vi "ScopeIntegrateSignal.vi"() -> ()   [LabVIEW 2018]
doc: "This example illustrates how to use autosetup and continuously acquires waveforms from a single channel using the following steps:\n\n1. Specify a valid VISA session. \n2. Specify a channel. \n3. Specify a time-out value for reading waveform.\n4. Run the VI. The graph displays the waveform you acquire."
uses:
  <vilib>/Analysis/baseanly.llb/Mean (DBL).vi
  <vilib>/Analysis/8numeric.llb/1D Numeric Integration.vi
  <instrlib>/Tektronix DPO MSO 2000 4000 Series/Public/Data/Read (Single Waveform).vi
  <instrlib>/Tektronix DPO MSO 2000 4000 Series/Tektronix DPO MSO 2000 4000 Series.lvlib
  <vilib>/Analysis/NI_AALPro.lvlib
  <vilib>/Analysis/NI_AALBase.lvlib
panel:
  out "Numeric":i32=1328
  out "standard deviation":dbl=1.3029024695657787 format="%0.2f"
  out "mean":dbl=2.2899697361108426 format="%0.2f"
  in  "Looping?":bool=TRUE
  in  "stop":bool
  out "integrated signal array":dbl[](array[numeric])=[0.18384399999980483, 1.0317809999998684, 1.3195783888887622, 2.3158365555554963, 0.04278729777806473, 1.1630631999997754, 3.3124563999997245, 3.497783541110766, 3.1549023744437497, 3.755903906666071, 3.3056046966661468, 3.106938013333607, 2.0850505944443567, 0.7116690033303827, 0.3406699844465184, 0.2005544977782775, 0.8526708144434995, 17.02474333444437, 1.3222985777702674, 1.0146186222293065, 0.6997047444517787, 1.2871290444375227, 20.821349922229718, 0.5246940888823304, 2.799625122228476, 1.648999088882956, 0.1761865444374138, 1.4400063555625282, 0.4872134555622556, 0.182366488894913, 0.13585464445012588, 1.4629045222283865, 1.8308287333288202, 1.3392077333367414, 2.7180222222237846, 1.4216097111038173, 0.2816763222150883, 0.3812891444506439, 2.365242422216168, 2.3021390333392304, 0.6825071333286256, 0.0959767555478045, 1.0579274000075247, 0.4138698333410148, 1.304622111118793, 0.49093292221467383, 0.9457530444370531, 101.81548561111937, 1.529317866658801, 0.33561907777122146, 1.0599211333392058, 0.8035876777852327, 0.5726897111173316, 0.06260372221603036, 2.2174570111179697, 0.5724496666644885, 0.5157550999971418, 2.8346701888819488, 2.778916566673187, 0.765314000007485, 0.9394557555628589, 0.6897417333308761, 3.7532666666722387, 2.173821266666129, 0.4845779333312618, 1.060541600000534, 2.2861999333331147, 0.11699586666738315, 0.9563122888909481, 1.8866587555542365, 2.7708600444424665, 3.598289155551745, 1.7618008444416102, 1.1966221111136597, 2.265614066664132, 0.20330315555749479, 0.12547351111451932, 0.3422101111106736, 0.5313641333342627, 1.0522981555572077, 0.3378435777794101, 2.006787177780507, 2.1922246888884085, 3.361183577780303, 0.6140928222222171, 1.4745631555535357, 0.3275447555555265, 0.6753259555530603, 2.815404511113747, 0.44156842222977544, 1.689486888890445, 1.640821333334569, 2.9290531555559047, 0.6118766222224593, 151.72732157777253, 0.826040555558351, 2.2798071111146094, 0.36612853333442347, 1.370790888899429, 2.277512288885853, 2.583507888883297, 0.5587739999998309, 1.7333380222304962, 0.9870752666637039, 0.14599966667146197, 1.835137177779994, 0.23406471110102162, 0.49785124444643347, 0.5946523500004227, 0.07523338888929976, 0.5758768055563855, 0.0733093944444089, 0.359282266667846, 0.010280066666889544, 0.681827916665766, 0.3919141444447414, 0.12973324444464956, 0.6164764222229102, 0.3204300611109303, 0.0720933000008443, 0.12928820555576342, 0.6098657666660594, 0.11357656111182071, 0.26238870555593635, 0.37584263333213874, 0.2554021388892921, 0.20303043333085263, 0.3101077888884636, 0.35926910555497565, 0.00022648888919396017, 0.26812556111169467, 0.10511678333299901, 0.5440186111114619, 0.01743401111172833, 0.3281956277780249, 0.8202786388912735, 0.3696199722241836, 0.04841992222217021, 0.3239199111107238, 0.3001403277771748, 0.08190676111082815, 0.40686790555485663, 86.0430172333338, 0.0016486000007947049, 0.14501810000032683, 0.3358190111111883, 0.030844705554956643, 0.5548646833340989, 0.3074427111109858, 0.1855340222226348, 0.0023650388895090843, 0.5550829666656036, 0.3319229277786019, 0.2979634833328052, 0.6956377888881221, 0.4173154666666514, 0.6801122888883514, 0.139358950000252, 0.2027275388881625, 0.4752827277773105, 0.06920137222224754, 0.1462285888899195, 0.3104269499993294, 0.6071250944441561, 0.15783686666638486, 0.3827724055561009, 0.024903588888977986, 0.9917656444440512, 0.250505066669551, 0.10083276666760904, 0.37267306666646277, 0.34872057222288716, 0.5987366722238008, 0.6558884666666526, 0.0029425500005292034, 1.4289747000062263, 1.077603833340331, 0.2976313222159524, 0.16553077777104885, 0.04071188888223318, 0.6158996666579656, 0.6296267222305018, 0.0043566777700086495, 2.304217255548706, 1.149385477774478, 0.37190994443622916, 1.321093977771371, 0.8237574666736233, 0.4398182000074706, 0.34472841110549224, 101.6373810333415, 0.842691444459666, 4.352914222217547, 3.4642069999796674, 0.6703112222367144, 1.9725337222045751, 3.6376435555696567, 3.5489517222082103, 6.32480072220843, 6.1287116110974, 1.546892722234429, 5.2348347777493744, 1.0970715000174573, 6.749840833347956, 9.231031055566662, 3.8409967777967826, 1.4225064444326108, 2.374212277792598, 4.324341611124469, 2.3102265555462838, 5.294125333340804, 6.662379777792693, 1.101190333327366, 5.148103777766739, 11.361353666678252, 5.932165388874546, 8.079377111096475, 5.080487277791736, 7.687094111125154, 0.3043856111193732, 10.670411777788116, 10.065965944451424, 0.5244318333399753, 13.074301777792584, 5.415608833316831, 1.9877505555598742, 1.3460380222320463, 0.5223974444430709, 2.1154885555578624, 2.5680954444446416, 1.317197888891957, 1.7756387999954955, 0.6476903333353883, 2.000213466674835, 0.0013438888889201112, 0.6318706222236417, 0.3013760666611618, 25.54041106667208, 0.3399827111113684, 0.16931690555602244, 0.3304252166661164, 0.16594397222185006, 0.12300538333289182, 0.2824761944441453, 0.17886768888885446, 0.6391234222220713, 0.3861981777783553, 0.09919301111110637, 0.2602778944443442, 0.13828761666639436, 0.1439515499997701, 0.3348733555558696, 0.06759907222323568, 0.5780929555568003, 0.24132427777802898, 0.04788488333396096, 0.3549457666659056, 0.3813597611109805, 0.11640393888960737, 0.5092426666667609, 0.13405288888820138, 14.625359033335016, 0.05221748888888154, 0.31403203888894826, 0.6693128444436998, 0.005222283332966806, 0.3896295277778545, 0.7952144388883583, 0.24450921666717135, 0.5297790777771815, 0.20670765000030916, 0.5681828666660081, 0.1069472055550931, 0.13426145555557506, 0.3312466500002883, 0.43531609444513375, 0.11154298888868011, 0.2259397222227168, 0.1524273555549207, 0.24677374444440603, 0.09216521111142176, 0.3101080833340964, 0.22031912777769935, 0.2475422000001521, 1.3618345499998947, 17.445979400003228, 16.615822750000493, 0.4773475000002133, 0.3393787500008643, 0.04931600000073315, 0.12953424999985447, 0.28308700000064296, 0.19237174999942008, 0.5199734999998644, 0.142788500000246, 0.33203175000057883, 0.4310394999999665, 0.3645760000005205, 0.06618225000005556, 0.44678924999943687, 0.024376499999411837, 0.20625500000275016, 0.08267749999828847, 0.22802799999867632, 0.07276249999920412, 0.44335200000030284, 0.0496382499990714, 0.5315962500021181, 0.06361550000044675, 0.17397174999885656, 0.5269249999999596, 0.2847330000002843, 0.14892249999982873, 0.06833175000003813, 0.00407175000068912, 0.4706767500019842, 0.1931362500003876, 0.24743474999997855, 0.3267587499997586, 0.0032507499995494214, 0.32125324999951416, 0.10164150000049926, 0.7838847499994154, 0.008091750000458654, 0.2176699999993266, 0.07650324999973851, 0.0022212500027330006, 0.041141250000310076, 0.1489822500003326, 0.2168092500004909, 0.16538550000185726, 0.08536075000076164, 0.190122249999861, 0.5998322500008049, 28.680398000002064, 0.6187474999993525, 0.08531399999973999, 0.08160100000009078, 0.6139035000013131, 0.08930725000039622, 0.1450710000001851, 0.4101759999997813, 0.35099600000022385, 0.36297850000029674, 0.4592644999999577, 0.25403500000172463, 0.0867375000007252, 0.2453322500000547, 0.1944042499998531, 0.018714750000023997, 0.37648899999931185, 0.012715000001591602, 0.1927334999993482, 0.15977174999992297, 0.5291257500000134, 0.37876350000072223, 0.23590874999947117, 0.05364799999968502, 0.04620049999988192, 0.08524850000111968, 0.028889750000128188, 0.336404500000131, 0.3814829999994586, 0.2656415000005441, 0.410605249998843, 0.037172999999793066, 0.26168800000125964, 20.260669000001442, 0.08019799999975162, 0.7069057500003919, 0.31472775000048986, 0.37307899999986394, 0.0110565000000994, 0.13501024999991432, 0.14727929999999934, 0.21339299999999023, 0.02721419999992087, 0.07464689999991106, 0.14395890000017095, 0.34344930000013324, 0.015313399999842832, 0.6588593000001416, 0.4972851000002087, 0.3576490000000021, 11.11897150000153, 0.8618529000002184, 0.5242404000001161, 0.16577289999988945, 0.2920685000003668, 0.12882070000117896, 0.1572200000005631, 0.2500369000004453, 0.23411990000015606, 0.11932270000000361, 0.08258360000011962, 0.13107790000048297, 0.10625830000042791, 0.24169929999949188, 0.181091700000621, 0.4045321000002707, 0.02549239999981485, 11.009053400001747, 0.5185025000002534, 0.25739325000127444, 0.5570394999992666, 0.386703250000732, 0.1552977500026714, 0.13306025000053684, 0.417687499999696, 0.6744872499992, 0.05852224999985313, 0.052378749999716236, 0.445232749999383, 0.5410842500004203, 0.20523499999993644, 0.2801555000000188, 0.06528799999911802, 0.01569175000001492, 0.06526225000005668, 0.32613749999987174, 0.04233049999922371, 0.4633337500004067, 0.5337992500000113, 0.43712474999990336, 0.4483537500005218, 0.35557375000009217, 0.10384350000047002, 0.24243200000000584, 0.40484274999987835, 0.143242000000006, 0.09111275000002417, 0.414716500000291, 0.0770889999993702, 0.36445474999995975, 0.4802162500000841, 0.19453125000067867, 0.33064724999990525, 0.014332499998676754, 0.07840850000000014, 0.4524680000002277, 0.3138670000003037, 0.08756499999993521, 0.3209355000014753, 0.4538340000006271, 0.15107975000056043, 0.13949374999992112, 0.01167050000059417, 0.3515565000003138, 28.02954674999923]
  out "bkgd":dbl=0.0001912722222221193 format="%0.4f"
  out "bkgd stop":dbl=0.00015854545454545456
  out "bkgd start":dbl=1.4545454545454546e-05
  out "dt":dbl=4e-10
  out "error":i32
  out "integral (nVs)":sgl=28.0
  out "stop int":dbl=0.00019972727272727273
  out "start int":dbl=0.00019787272727272726
  in  "Channel (0: Channel 1)":u16(ring)=2 items=["Channel 1", "Channel 2", "Channel 3", "Channel 4", "Math", "Reference 1", "Reference 2", "Reference 3", "Reference 4"]
  in  "Maximum Time (10000ms)":u32=10000
  in  "VISA Resource Name":refnum<visa-resource-name>="mdo4034c"
  out "Waveform Graph":waveform(dbl)(graph)={"t0"=timestamp(-0.00019704399999997957 s since 1904-01-01), "dt"=4e-10, "Y"=array[1000000 elements]}
  # "(C) 2006 - 2022. National Instruments Corporation. ALL RIGHTS RESERVED."
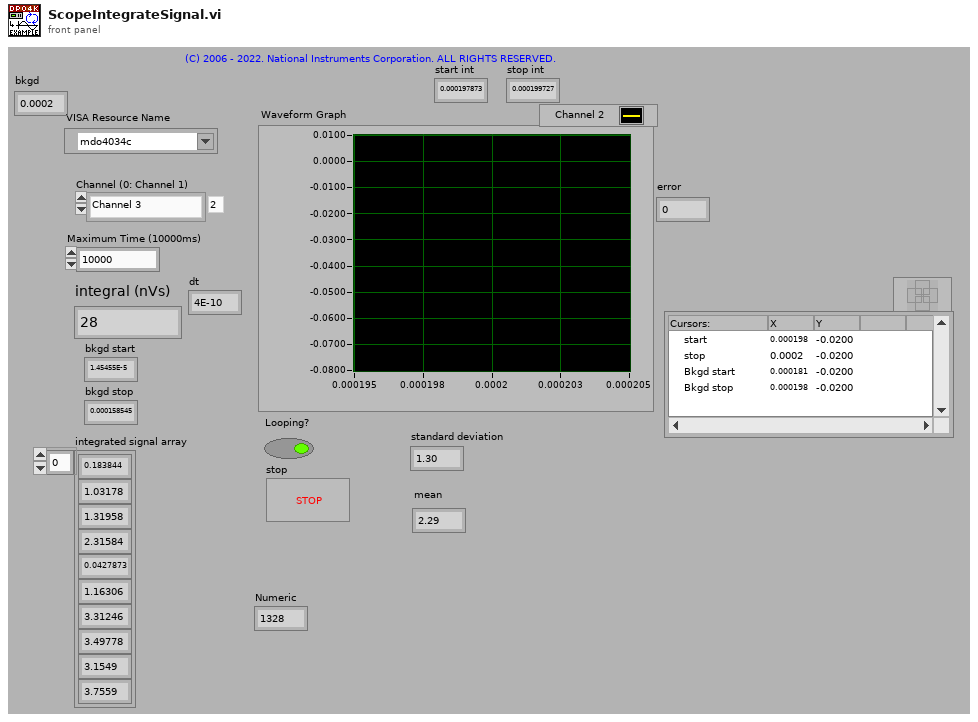
[diagram p1: front panel]
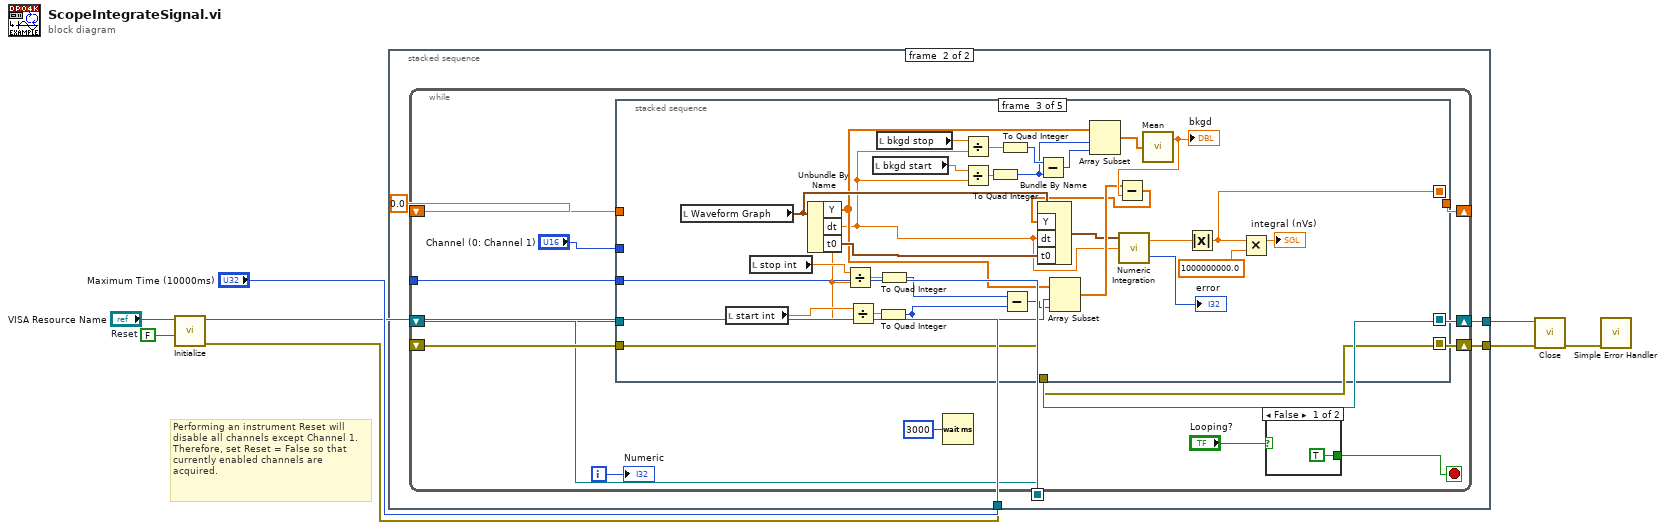
[diagram p0: block diagram]
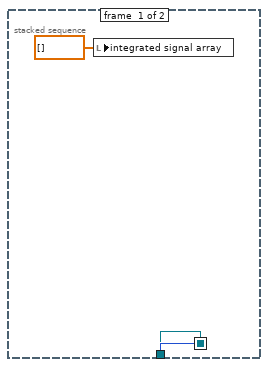
[diagram p2: hidden frame]
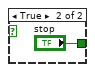
[diagram p3: hidden frame]
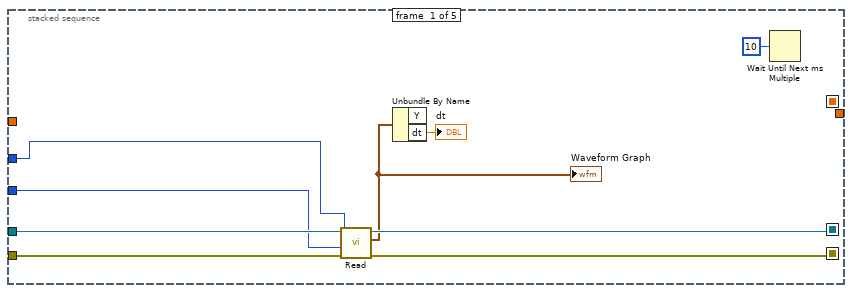
[diagram p4: hidden frame]
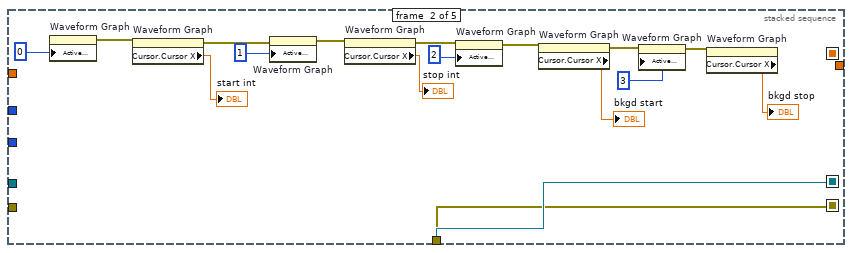
[diagram p5: hidden frame]
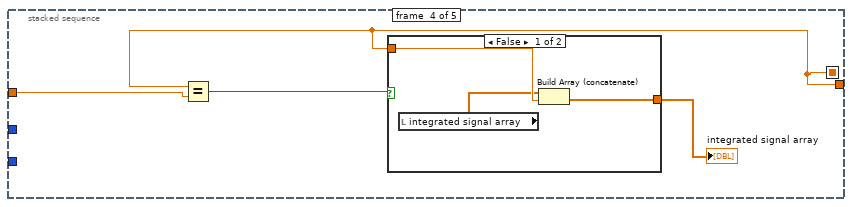
[diagram p6: hidden frame]
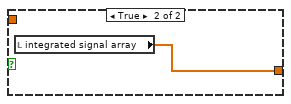
[diagram p7: hidden frame]
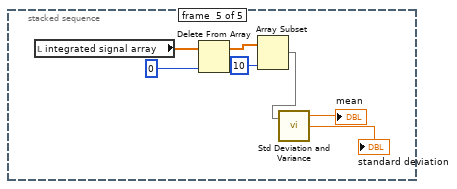
[diagram p8: hidden frame]
diagram:
  w4 = FALSE  # Reset
  # "Performing an instrument Reset will disable all channels except Channel 1. Therefore, set Reset = False so that currently enabled channels are acquired."
  n1 = call <instrlib>:"Initialize.vi"("Reset (True)"=w4, "VISA resource name"="VISA Resource Name") -> ("error out"=w2:errorcluster, "VISA resource name out"=w1:refnum<visa-resource-name>)  [unwired: 8 in]
  n2 = stacked-sequence {
    seq-local: [w12 _] -> [_ w16]
    seq-local: [w11 _] -> [_ w15]
    seq-local: [w10 _] -> [_ w14]
    tunnel: "Maximum Time (10000ms)" -> [w12 _]
    tunnel: w2 -> [w11 _]
    tunnel: w1 -> [w10 _]
    tunnel: [_ w18] -> w7
    tunnel: [_ w17] -> w6
    frame #0 {
      n3 = local write "integrated signal array"(dbl[] [] ("integrated signal array")) -> ()
    }
    frame #1 {
      n4 = while {
        tunnel: w16 -> [w28]
        shift-right: [w29] -> w17
        shift-left: w15 -> [w27]
        shift-right: [w30] -> w18
        shift-left: w14 -> [w26]
        shift-right: [w25] -> _
        shift-left: 0.0 -> [w24]
        i -> [w21]
        stop <- w22 stop-if-true
        n5 = stacked-sequence {
          seq-local: [w39 _ _ _ _] -> [_ w58 _ _ _]
          seq-local: [w37 _ _ _ _] -> [_ w57 _ _ _]
          seq-local: [_ _ w62 _ _] -> [_ _ _ w88 _]
          tunnel: w26 -> [w41 _ _ _ _]
          tunnel: w27 -> [w40 _ _ _ _]
          tunnel: w28 -> [w36 _ _ _ _]
          tunnel: "Channel (0: Channel 1)" -> [w34 _ _ _ _]
          tunnel: [_ w58 _ _ _] -> w30
          tunnel: [_ w57 _ _ _] -> w29
          tunnel: [_ _ _ w88 _] -> w25
          tunnel: w24 -> [_ _ _ w87 _]
          frame #0 {
            n6 = call-poly <instrlib>:"Read.vi"("error in (no error)"=w40, "Maximum Time (10000ms)"=w36, "Channel (0: Channel 1)"=w34, "VISA resource name"=w41) -> ("error out"=w37:errorcluster, "Waveform Graph"=w33:waveform(dbl), "VISA resource name out"=w39:refnum<visa-resource-name>)  [unwired: 5 in]
            "Waveform Graph" <- w33
            n7 = Unbundle By Name(w33) -> ("dt"=→"dt":dbl)  [unwired: 1 out]
            n8 = Wait Until Next ms Multiple(millisecond multiple=u32 10) -> ()  [unwired: 1 out]
          }
          frame #1 {
            n9 = property on="Waveform Graph" class="WFGraph (strict)"("Active Cursor"=0 ("Cursor.Cursor Index")) -> (error out=w55:errorcluster)  [unwired: 2 in, 1 out]
            n10 = property on="Waveform Graph" class="WFGraph (strict)"(error in=w55) -> (error out=w54:errorcluster, "Cursor.Cursor X"=→"start int":dbl)  [unwired: 1 in, 1 out]
            n11 = property on="Waveform Graph" class="WFGraph (strict)"(error in=w54, "Active Cursor"=1 ("Cursor.Cursor Index")) -> (error out=w53:errorcluster)  [unwired: 1 in, 1 out]
            n12 = property on="Waveform Graph" class="WFGraph (strict)"(error in=w53) -> (error out=w48:errorcluster, "Cursor.Cursor X"=→"stop int":dbl)  [unwired: 1 in, 1 out]
            n13 = property on="Waveform Graph" class="WFGraph (strict)"(error in=w48, "Active Cursor"=u32 2) -> (error out=w49:errorcluster)  [unwired: 1 in, 1 out]
            n14 = property on="Waveform Graph" class="WFGraph (strict)"(error in=w49) -> (error out=w45:errorcluster, "Cursor.Cursor X"=→"bkgd start":dbl)  [unwired: 1 in, 1 out]
            n15 = property on="Waveform Graph" class="WFGraph (strict)"(error in=w45, "Active Cursor"=u32 3) -> (error out=w46:errorcluster)  [unwired: 1 in, 1 out]
            n16 = property on="Waveform Graph" class="WFGraph (strict)"(error in=w46) -> ("Cursor.Cursor X"=→"bkgd stop":dbl)  [unwired: 1 in, 2 out]
          }
          frame #2 {
            n17 = local read "Waveform Graph"() -> (w77:waveform(dbl))
            n18 = local read "start int"() -> (w85:dbl)
            n19 = local read "stop int"() -> (w86:dbl)
            n20 = Unbundle By Name(w77) -> ("Y"=w75:dbl[], "dt"=w59:dbl, "t0"=w76:timestamp)
            n21 = Divide(x=w86, y=w59) -> (x/y=w84:dbl)
            n22 = Divide(x=w85, y=w59) -> (x/y=w83:dbl)
            n23 = local read "bkgd start"() -> (w71:dbl)
            n24 = local read "bkgd stop"() -> (w72:dbl)
            n25 = To Quad Integer(1:w83) -> (0:w81:i64)
            n26 = To Quad Integer(1:w84) -> (0:w82:i64)
            n27 = Divide(x=w72, y=w59) -> (x/y=w73:dbl)
            n28 = Divide(x=w71, y=w59) -> (x/y=w74:dbl)
            n29 = To Quad Integer(1:w74) -> (0:w68:i64)
            n30 = To Quad Integer(1:w73) -> (0:w70:i64)
            n31 = Subtract(x=w82, y=w81) -> (x-y=w80:i64)
            n32 = Subtract(x=w70, y=w68) -> (x-y=w69:i64)
            n33 = Array Subset(array=w75, index=w81, length=w80) -> (w65:dbl[])
            n34 = Array Subset(array=w75, index=w68, length=w69) -> (w67:dbl[])
            n35 = call-poly <vilib>:"Mean.vi"("X"=w67) -> ("mean"=w66:dbl)  [unwired: 1 out]
            "bkgd" <- w66
            n36 = Subtract(x=w65, y=w66) -> (x-y=w63:dbl[])
            n37 = Bundle By Name(cluster=w77, "Y"=w63, "dt"=w59, "t0"=w76) -> (w64:waveform(dbl))
            n38 = call-poly <vilib>:"Numeric Integration.vi"("dt"=w59, "Input Array"=w64) -> ("error"=→"error":i32, "result"=w79:dbl)  [unwired: 1 in]
            n39 = Absolute Value(x=w79) -> (abs(x)=w62:dbl)
            n40 = Multiply(x=w62, y=1000000000.0) -> (x*y=→"integral (nVs)":dbl)
          }
          frame #3 {
            n41 = Equal?(x=w88, y=w87) -> (x = y?=w90:bool)
            n42 = case shown="False" w90 {
              tunnel: w88 -> [w93 _]
              tunnel: [w92 w94] -> w89
              frame False {
                n43 = local read "integrated signal array"() -> (w91:dbl[])
                n44 = Build Array (concatenate)(w91, w93) -> (w92:dbl[])
              }
              frame True {
                n45 = local read "integrated signal array"() -> (w94:dbl[])
              }
            }
            "integrated signal array" <- w89
          }
          frame #4 {
            n46 = local read "integrated signal array"() -> (w101:dbl[])
            n47 = Delete From Array(array=w101, index=0) -> (array with subset deleted=w97:dbl[])  [unwired: 1 in, 1 out]
            n48 = Array Subset(array=w97, length=10) -> (w96:dbl[])  [unwired: 1 in]
            n49 = call <vilib>:"Std Deviation and Variance.vi"("X"=w96) -> ("mean"=→"mean":dbl, "standard deviation"=→"standard deviation":dbl)  [unwired: 1 in, 1 out]
          }
        }
        n50 = Wait (ms)(milliseconds to wait=u32 3000) -> ()  [unwired: 1 out]
        n51 = case shown="False" "Looping?" {
          tunnel: [TRUE ("stop") "stop"] -> w22
          frame False {
          }
          frame True {
          }
        }
        "Numeric" <- w21
      }
    }
  }
  n52 = call <instrlib>:"Close.vi"("error in (no error)"=w6, "VISA resource name"=w7) -> ("error out"=w5:errorcluster)  [unwired: 9 in]
  n53 = call <vilib>:"Simple Error Handler.vi"("error in (no error)"=w5) -> ()  [unwired: 4 in, 5 out]
